vi "DataAcquisition1.vi"(0 "Handle In":i32, 1 "LP1 Pin":u16, 5 "Solenoid Supply Pin":u16=5, 7 "LabJack Supply Pin":u16=7, 9 "Relay Supply Pin":u16=9, 11 "error in":errorcluster, 12 "k":dbl) -> (2 "LP1 Voltage Reading":dbl, 3 "Displacement Reading [meter]":dbl, 4 "Thrust Reading [Newton]":dbl, 6 "Solenoid Supply Voltage":dbl, 8 "LabJack Supply Voltage":dbl, 10 "Relay Supply Voltage":dbl, 15 "error out":errorcluster[](array[cluster]))   [LabVIEW 2021]
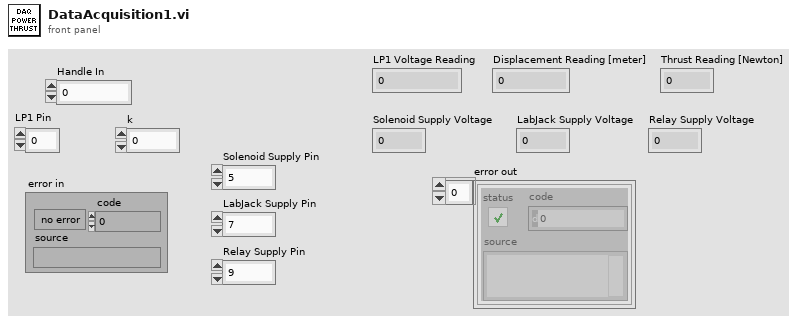
[diagram p1: front panel]
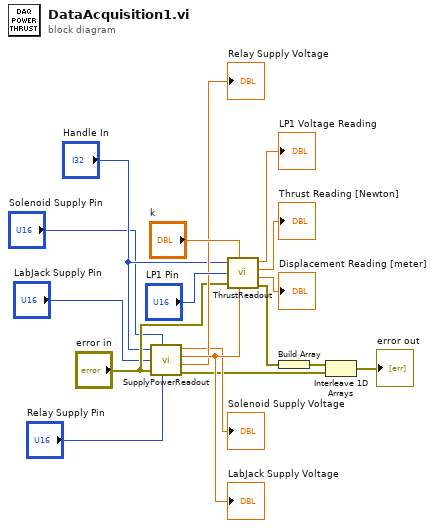
[diagram p0: block diagram]
diagram:
  n1 = call "SupplyPowerReadout.vi"("Handle In"="Handle In", "Solenoid Supply Pin"="Solenoid Supply Pin", "LabJack Supply Pin"="LabJack Supply Pin", "error in"="error in", "Relay Supply Pin"="Relay Supply Pin") -> ("Solenoid Supply Voltage"=→"Solenoid Supply Voltage":dbl, "LabJack Supply Voltage"=w17:dbl, "Relay Supply Voltage"=→"Relay Supply Voltage":dbl, "error out"=w7:errorcluster[])
  "LabJack Supply Voltage" <- w17
  n2 = call "ThrustReadout.vi"("Handle In"="Handle In", "k"="k", "LP1 Pin"="LP1 Pin", "error in"="error in", "LabJack Supply"=w17) -> ("Voltage Reading"=→"LP1 Voltage Reading":dbl, "Thrust Reading [Newton]"=→"Thrust Reading [Newton]":dbl, "Displacement Reading [meter]"=→"Displacement Reading [meter]":dbl, "error out"=w5:errorcluster)
  n3 = Build Array(w5) -> (w6:errorcluster[])
  n4 = Interleave 1D Arrays(w6, w7) -> (→"error out":errorcluster[])
